vi "sub vi - PowerSpectrum 2.vi"(6 "filename":string, 8 "number of samples per channel":i32=60000, 9 "rate (Hz)":dbl=20000.0 format="%0.2f", 10 "Save Raw Data":bool, 11 "Axis  2":u16(ring) items=["QPD2", "QPD1"]) -> (3 "?":waveform(dbl)[](graph))   [LabVIEW 2010]
uses:
  <vilib>/DAQmx/read.llb/DAQmx Read (Analog 1D Wfm NChan NSamp).vi
  <vilib>/DAQmx/create/channels.llb/DAQmx Create Channel (AI-Voltage-Basic).vi
  <vilib>/DAQmx/configure/timing.llb/DAQmx Timing (Sample Clock).vi
  <vilib>/daqmx/miscellaneous.llb/DAQmx Fill In Error Info.vi
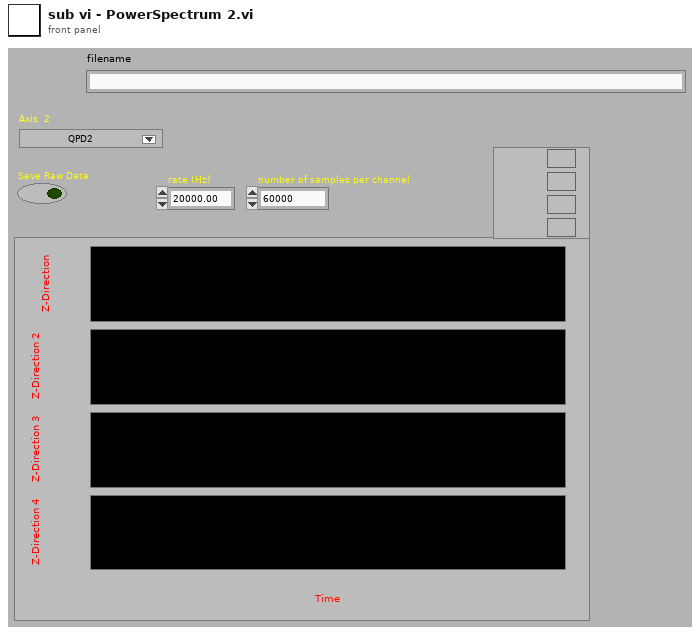
[diagram p1: front panel]
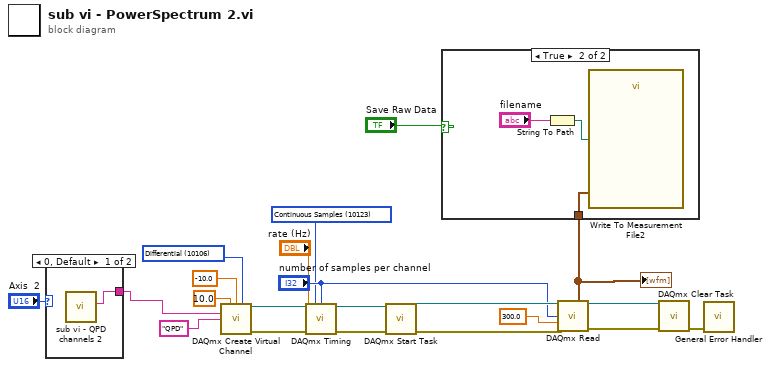
[diagram p0: block diagram]
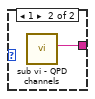
[diagram p2: hidden frame]
diagram:
  w8 = 10123 items=["Finite Samples"=10178, "Continuous Samples"=10123, "Hardware Timed Single Point"=12522] ("sample mode")
  w15 = 10106 items=["default"=-1, "RSE"=10083, "NRSE"=10078, "Differential"=10106, "Pseudodifferential"=12529] ("input terminal configuration")
  n1 = case shown="0, Default" "Axis  2" {
    tunnel: [w22 w23] -> w1
    frame 0, Default {
      n2 = call "sub vi - QPD channels 2.vi"() -> ("QPD Channels"=w22:tag)  [unwired: 1 in, 9 out]
    }
    frame 1 {
      n3 = call "sub vi - QPD channels.vi"() -> ("QPD Channels"=w23:tag)  [unwired: 11 out]
    }
  }
  n4 = call-poly <vilib>:"DAQmx Create Virtual Channel.vi"("maximum value"=10.0, "minimum value"=-10.0, "input terminal configuration"=w15, "physical channels"=w1, "name to assign"="QPD") -> ("task out"=w14:refnum<k21>, "error out"=w11:errorcluster)  [unwired: 4 in, 5 out]
  n5 = call-poly <vilib>:"DAQmx Timing.vi"("task/channels in"=w14, "sample mode"=w8, "samples per channel"="number of samples per channel", "rate"="rate (Hz)", "error in"=w11) -> ("task out"=w13:refnum<k21>, "error out"=w12:errorcluster)  [unwired: 2 in, 7 out]
  n6 = call <vilib>:"DAQmx Start Task.vi"("task/channels in"=w13, "error in"=w12) -> ("task out"=w17:refnum<k21>, "error out"=w16:errorcluster)  [unwired: 12 out]
  n7 = call-poly <vilib>:"DAQmx Read.vi"("task/channels in"=w17, "number of samples per channel"="number of samples per channel", "timeout"=300.0, "error in"=w16) -> ("task out"=w19:refnum<k21>, "data"=w3:waveform(dbl)[], "error out"=w18:errorcluster)  [unwired: 9 out]
  "?" <- w3
  n8 = case shown="True" "Save Raw Data" {
    tunnel: w3 -> [_ w26]
    frame False {
    }
    frame True {
      n9 = String To Path(string="filename") -> (path=w25:path)
      n10 = call "Write To Measurement File2"("Signals"=w26, "Filename"=w25) -> ()  [unwired: 15 in, 3 out]
    }
  }
  n11 = call <vilib>:"DAQmx Clear Task.vi"("task in"=w19, "error in"=w18) -> ("error out"=w20:errorcluster)  [unwired: 13 out]
  n12 = call <vilib>:"General Error Handler.vi"("error in (no error)"=w20) -> ()  [unwired: 1 in, 14 out]
